vi "MultiDepth ILC Homing.vi"(7 "Offset Home 2 RCM":dbl[](array[numeric])=[0.0, 0.0, 0.0, 0.0], 8 "error in":errorcluster, 9 "Stage PID Cluster":T2={"Stage Z PID"={"Kp"=0.0005, "Kd"=0.001, "Ki"=0.0}, "Stage Y PID"={"Kp"=0.0003, "Kd"=0.01, "Ki"=0.0}, "Stage X PID"={"Kp"=0.0003, "Kd"=0.01, "Ki"=0.0}}, 10 "L1 to L4 PID Cluster":T1={"L1 PID Gains"={"Kp"=0.005, "Kd"=0.5, "Ki"=0.0005}, "L2 PID Gains"={"Kp"=0.01, "Kd"=1.0, "Ki"=0.005}, "L3 PID Gains"={"Kp"=0.05, "Kd"=1.0, "Ki"=0.0005}, "L4 PID Gains"={"Kp"=0.1, "Kd"=0.1, "Ki"=0.0005}}, 11 "FPGA VI Reference In":refnum<k20>) -> (0 "error out":errorcluster, 1 "Last Stage Posit":dbl[](array[numeric]), 2 "Last L1 to L4 Posit":dbl[](array[numeric]), 3 "FPGA VI Reference Out":refnum<k20>)   [LabVIEW 2016]
uses:
  <vilib>/Platform/TimedLoop/XDataNode/timing_clust.ctl
  <vilib>/Platform/TimedLoop/XDataNode/nitl_modes.ctl
  <vilib>/Platform/TimedLoop/XDataNode/wakeup.ctl
  Library/KevinLibraryAll/labview2010/kevLib2010/Simple Filters/kDelay.vi
  Global Variables.vi
  <vilib>/Utility/error.llb/Error Cluster From Error Code.vi
  <vilib>/rvi/errors/niLvFpgaAdjustHostInterfaceError.vi
  <vilib>/platform/TimedLoop/XDataNode/XDataNode.xnode
  <vilib>/rvi/interface/nirviReadWriteControl/nirviReadWriteControl.xnode
  FPGA Bitfiles/PhantomControlPI_FPGATarget_QuadCtr2_E2412E44.lvbitx
  IRISS_FPGA_IO.vi
  <vilib>/Platform/TimedLoop/XDataNode/XDNodeRunTimeDep.lvlib
  Library/KevinLibraryAll/labview2010/kevLib2010.lvlib
  Library/KevinLibraryAll/labview2011/kevLib2011.lvlib
  Library/KevinLibraryAll/labview/KevLib01.lvlib
  Library/jmslib.lvlib
  NiFpgaLv.dll
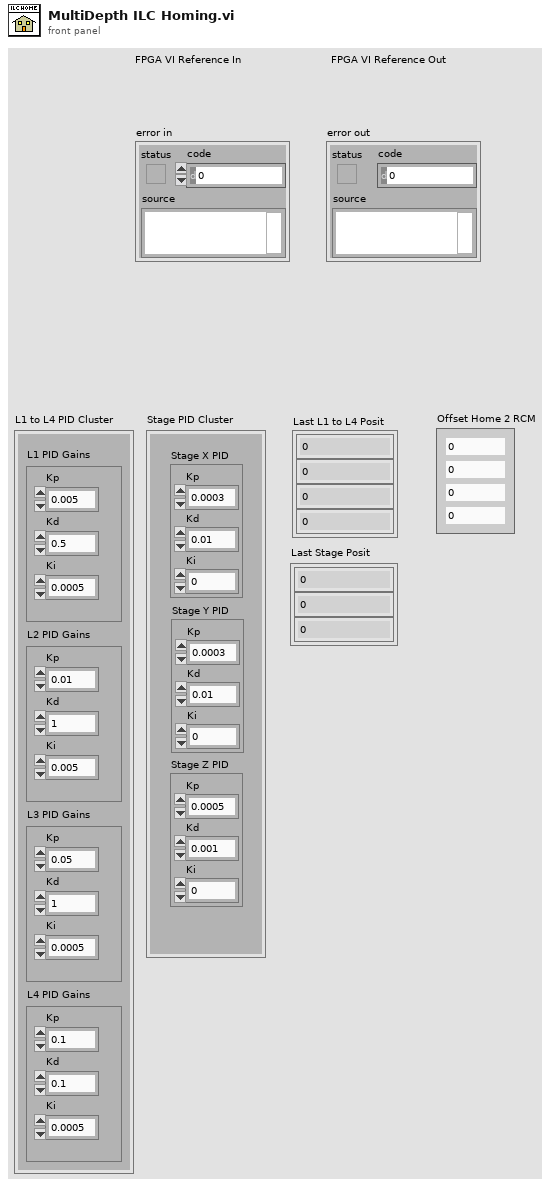
[diagram p1: front panel]
types:
  T1 = cluster{"L1 PID Gains":cluster{"Kp":dbl, "Kd":dbl, "Ki":dbl}, "L2 PID Gains":cluster{"Kp":dbl, "Kd":dbl, "Ki":dbl}, "L3 PID Gains":cluster{"Kp":dbl, "Kd":dbl, "Ki":dbl}, "L4 PID Gains":cluster{"Kp":dbl, "Kd":dbl, "Ki":dbl}}
  T2 = cluster{"Stage Z PID":cluster{"Kp":dbl, "Kd":dbl, "Ki":dbl}, "Stage Y PID":cluster{"Kp":dbl, "Kd":dbl, "Ki":dbl}, "Stage X PID":cluster{"Kp":dbl, "Kd":dbl, "Ki":dbl}}
  T3 = typedef "XDNodeRunTimeDep.lvlib/timing_clust.ctl" = cluster{"Expected End [f-1]":u64, "Actual End [f-1]":u64, "Finished Late? [f-1]":bool, "Expected End [i-1]":u64, "Actual End [i-1]":u64, "Finished Late? [i-1]":bool, "Expected Start [i]":u64, "Actual Start [i]":u64, "Expected Start [f]":u64, "Actual Start [f]":u64, "Source Name":string, "Structure Name":string, "Period":i64, "Deadline":i64, "Offset":i64, "Start":i64, "Priority":i32, "Timeout":i32, "Mode":T4, "Wakeup Reason":T5, "Error":errorcluster, "Source Type":string, "Secondary Source Type":string, "Global End Time":u64, "Global Start Time":u64, "Frame Duration":u64, "Iteration Duration":u64, "Assigned CPU":i32, "I/O Scan Engine Mode":u32}
  T4 = typedef "XDNodeRunTimeDep.lvlib/nitl_modes.ctl" = enum32{"No Change", "Process missed periods, maintain original phase", "Discard missed periods, maintain original phase", "Process missed periods, ignore original phase", "Discard missed periods, ignore original phase"}
  T5 = typedef "XDNodeRunTimeDep.lvlib/wakeup.ctl" = enum32{"Normal", "Aborted", "Asynchronous wakeup", "Timing source error", "Timed loop error", "Timeout"}
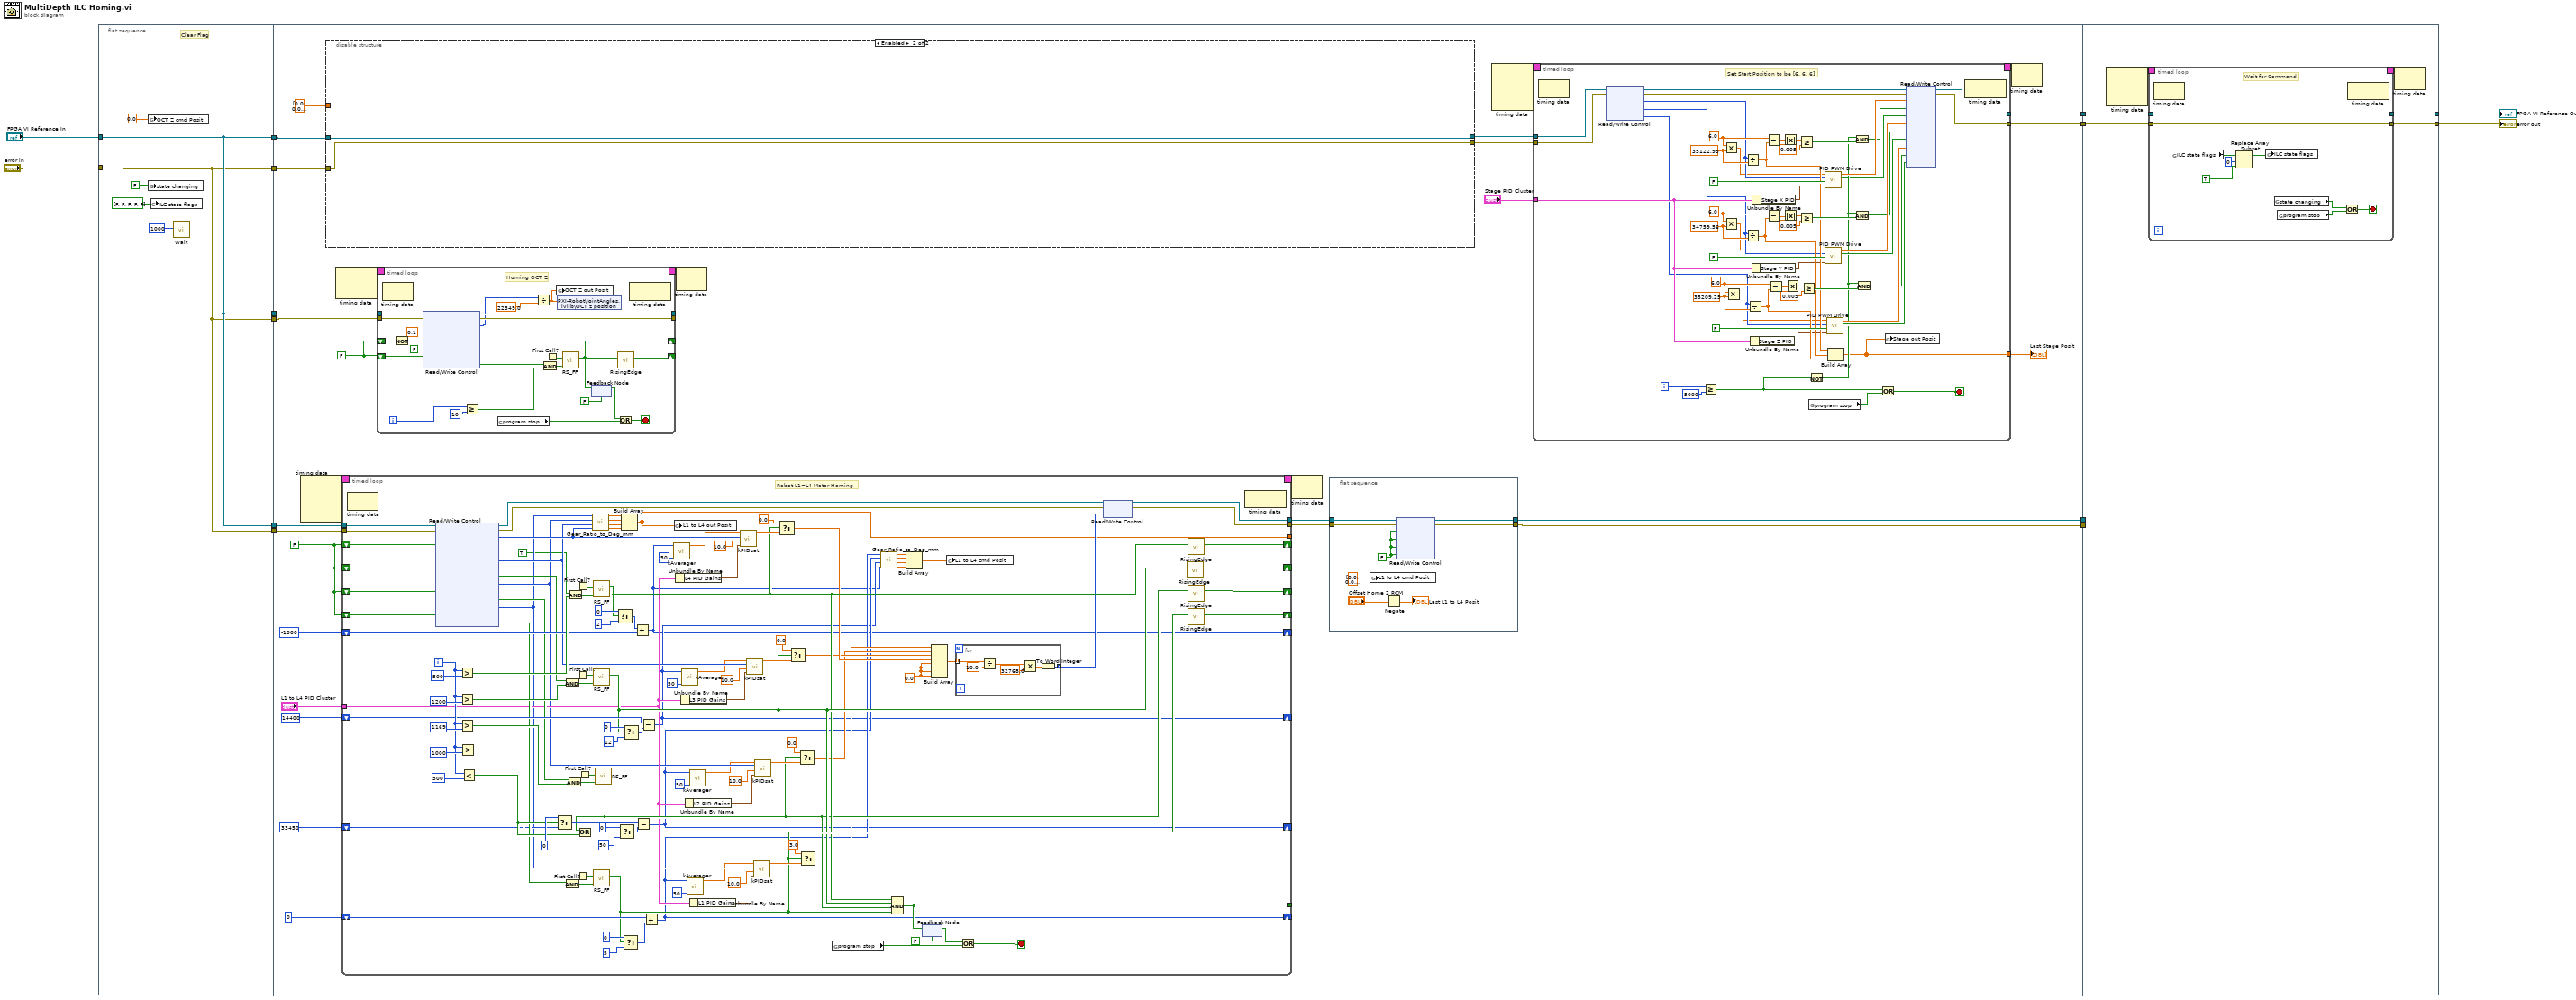
[diagram p0: block diagram]
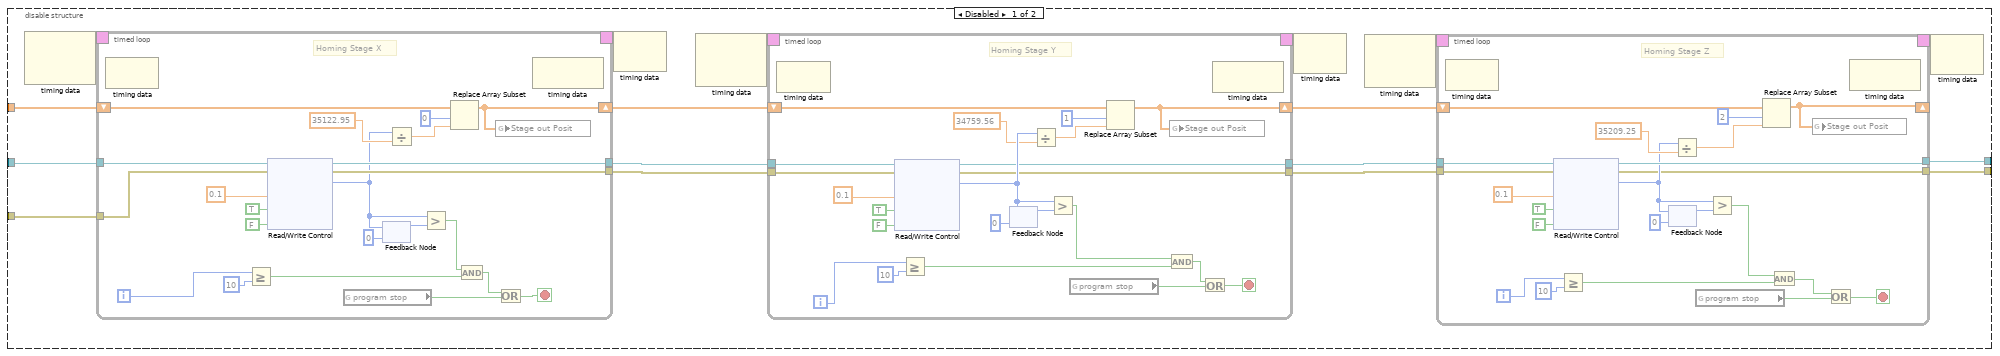
[diagram p2: hidden frame]
diagram:
  n1 = flat-sequence {
    tunnel: "FPGA VI Reference In" -> [w18]
    tunnel: "error in" -> [w17]
    tunnel: [w18] -> w14
    tunnel: [w18] -> w13
    tunnel: [w17] -> w12
    tunnel: [w17] -> w11
    tunnel: [w18] -> w6
    tunnel: [w17] -> w5
    tunnel: w14 -> [w48]
    tunnel: w13 -> [w47]
    tunnel: w12 -> [w46]
    tunnel: w11 -> [w45]
    tunnel: w6 -> [w42]
    tunnel: w5 -> [w41]
    tunnel: [w39] -> w4
    tunnel: [w38] -> w3
    tunnel: [w32] -> w2
    tunnel: [w31] -> w1
    tunnel: [w372] -> w8
    tunnel: [w371] -> w7
    tunnel: w4 -> [_]
    tunnel: w3 -> [_]
    tunnel: w2 -> [w370]
    tunnel: w1 -> [w369]
    frame #0 {
      # "Clear Flag"
      n2 = global write "Global Variables.vi" "OCT Z cmd Posit"(0.0) -> ()
      n3 = global write "Global Variables.vi" "state changing"(FALSE ("state changing")) -> ()
      n4 = global write "Global Variables.vi" "ILC state flags"(bool[] [FALSE, FALSE, FALSE, FALSE, FALSE]) -> ()
      n5 = call "Wait"("Count(mSec)"=u32 1000 ("milliseconds to wait")) -> ()  [unwired: 1 out]
    }
    frame #1 {
      w26 = FALSE ("Rising Edge")
      w40 = FALSE ("Rising Edge")
      n6 = node-c288() -> (w30:T3)  [unwired: 4 in]
      n7 = disable-structure shown="Enabled" {
        disable-tunnel: [w61 w147] -> w50
        disable-tunnel: [w60 w146] -> w49
        disable-tunnel: w48 -> [w59 w147]
        disable-tunnel: w46 -> [w58 w146]
        disable-tunnel: dbl[] [0.0, 0.0, 0.0] ("Stage Posit Array") -> [w51 _]
        frame Disabled {
          n8 = node-c288() -> (w63:T3)  [unwired: 2 in]
          n9 = timed-loop {
            timing: w63 -> [_]
            timing-out: [_] -> w62
            tunnel: w59 -> [w79]
            tunnel: w58 -> [w78]
            tunnel: [w77] -> w54
            tunnel: [w76] -> w53
            shift-right: [w68] -> w52
            shift-left: w51 -> [w70]
            i -> [w80]
            stop <- w73 stop-if-true
            # "Homing Stage X"
            n10 = node-c288() -> ()  [unwired: 1 in, 1 out]
            n11 = Greater Or Equal?(x=w80, y=10) -> (x >= y?=w89:bool)
            n12 = xnode "Read/Write Control"("FPGA VI Reference In"=w79, "error in"=w78, "X DC"=0.1 ("y"), "INHB X"=TRUE ("INHB Y"), "DIR X"=FALSE ("INHB Y")) -> ("FPGA VI Reference Out"=w77:refnum<k20>, "error out"=w76:errorcluster, "Position X"=w69:i32)
            n13 = global read "Global Variables.vi" "program stop"() -> (w75:bool)
            n14 = feedback #1(0 ("Position Y")) -> (w86:i32)
            n15 = feedback-in #1(w69) -> ()
            n16 = Divide(x=w69, y=35122.95) -> (x/y=w71:dbl)
            n17 = Greater?(x=w69, y=w86) -> (0:w87:bool)
            n18 = Replace Array Subset(array=w70, new element=w71, index=0) -> (w68:dbl[])
            n19 = And(x=w87, y=w89) -> (x .and. y?=w74:bool)
            n20 = global write "Global Variables.vi" "Stage out Posit"(w68) -> ()
            n21 = Or(x=w74, y=w75) -> (x .or. y?=w73:bool)
            n22 = node-c288() -> ()  [unwired: 1 in, 1 out]
          }
          n23 = node-c288(w62) -> ()  [unwired: 1 out]
          n24 = node-c288() -> (w65:T3)  [unwired: 2 in]
          n25 = timed-loop {
            timing: w65 -> [_]
            timing-out: [_] -> w64
            tunnel: w54 -> [w104]
            tunnel: w53 -> [w105]
            tunnel: [w102] -> w57
            tunnel: [w101] -> w56
            shift-right: [w94] -> w55
            shift-left: w52 -> [w95]
            i -> [w103]
            stop <- w100 stop-if-true
            # "Homing Stage Y"
            n26 = node-c288() -> ()  [unwired: 1 in, 1 out]
            n27 = xnode "Read/Write Control"("FPGA VI Reference In"=w104, "error in"=w105, "Y DC"=0.1 ("y"), "INHB Y"=TRUE, "DIR Y"=FALSE ("INHB Y")) -> ("FPGA VI Reference Out"=w102:refnum<k20>, "error out"=w101:errorcluster, "Position Y"=w112:i32)
            n28 = Greater Or Equal?(x=w103, y=10) -> (x >= y?=w115:bool)
            n29 = feedback #2(0 ("Position Y")) -> (w111:i32)
            n30 = feedback-in #2(w112) -> ()
            n31 = Divide(x=w112, y=34759.56) -> (x/y=w96:dbl)
            n32 = Greater?(x=w112, y=w111) -> (0:w113:bool)
            n33 = global read "Global Variables.vi" "program stop"() -> (w98:bool)
            n34 = Replace Array Subset(array=w95, new element=w96, index=1) -> (w94:dbl[])
            n35 = And(x=w113, y=w115) -> (x .and. y?=w99:bool)
            n36 = global write "Global Variables.vi" "Stage out Posit"(w94) -> ()
            n37 = Or(x=w99, y=w98) -> (x .or. y?=w100:bool)
            n38 = node-c288() -> ()  [unwired: 1 in, 1 out]
          }
          n39 = node-c288(w64) -> ()  [unwired: 1 out]
          n40 = node-c288() -> (w67:T3)  [unwired: 2 in]
          n41 = timed-loop {
            timing: w67 -> [_]
            timing-out: [_] -> w66
            tunnel: w57 -> [w141]
            tunnel: [w140] -> w61
            tunnel: w56 -> [w128]
            tunnel: [w127] -> w60
            shift-right: [w120] -> _
            shift-left: w55 -> [w121]
            i -> [w131]
            stop <- w125 stop-if-true
            # "Homing Stage Z"
            n42 = node-c288() -> ()  [unwired: 1 in, 1 out]
            n43 = xnode "Read/Write Control"("FPGA VI Reference In"=w141, "error in"=w128, "Z DC"=0.1 ("y"), "INHB Z"=TRUE ("INHB Y"), "DIR Z"=FALSE ("INHB Y")) -> ("FPGA VI Reference Out"=w140:refnum<k20>, "error out"=w127:errorcluster, "Position Z"=w133:i32)
            n44 = Greater Or Equal?(x=w131, y=10) -> (x >= y?=w129:bool)
            n45 = feedback-in #3(w133) -> ()
            n46 = feedback #3(0 ("Position Y")) -> (w134:i32)
            n47 = Divide(x=w133, y=35209.25) -> (x/y=w122:dbl)
            n48 = global read "Global Variables.vi" "program stop"() -> (w126:bool)
            n49 = Greater?(x=w133, y=w134) -> (0:w132:bool)
            n50 = Replace Array Subset(array=w121, new element=w122, index=2) -> (w120:dbl[])
            n51 = And(x=w132, y=w129) -> (x .and. y?=w124:bool)
            n52 = global write "Global Variables.vi" "Stage out Posit"(w120) -> ()
            n53 = Or(x=w124, y=w126) -> (x .or. y?=w125:bool)
            n54 = node-c288() -> ()  [unwired: 1 in, 1 out]
          }
          n55 = node-c288(w66) -> ()  [unwired: 1 out]
        }
        frame Enabled {
        }
      }
      n56 = node-c288() -> (w44:T3)  [unwired: 2 in]
      n57 = timed-loop {
        timing: w30 -> [_]
        timing-out: [_] -> w29
        tunnel: w47 -> [w262]
        tunnel: w45 -> [w261]
        shift-right: [w196] -> _
        shift-left: w26 -> [w260]
        shift-right: [w195] -> _
        shift-left: w26 -> [w259]
        shift-right: [w194] -> _
        shift-left: w26 -> [w258]
        shift-right: [w193] -> _
        shift-left: w26 -> [w257]
        shift-right: [w151] -> _
        shift-left: -1000 -> [w240]
        shift-right: [w152] -> _
        shift-left: 14400 -> [w232]
        shift-right: [w153] -> _
        shift-left: 33450 -> [w203]
        shift-right: [w154] -> _
        shift-left: 0 -> [w202]
        tunnel: [w197] -> _
        tunnel: [w177] -> w28
        tunnel: [w176] -> w27
        tunnel: "L1 to L4 PID Cluster" -> [w172]
        tunnel: [w150] -> _
        i -> [w242]
        stop <- w198 stop-if-true
        w188 = 0.0 ("element")
        # "Robot L1~L4 Motor Homing"
        n58 = node-c288() -> ()  [unwired: 1 in, 1 out]
        n59 = xnode "Read/Write Control"("FPGA VI Reference In"=w262, "error in"=w261, "Reset C1-4"=w260, "Reset C1-1"=w259, "Reset 3"=w258, "Reset 1"=w257) -> ("FPGA VI Reference Out"=w185:refnum<k20>, "error out"=w184:errorcluster, "32 bit Position C1-4"=w170:i32, "32 bit Position C1-1"=w169:i32, "Home L3"=w223:bool, "32 bit Position 3"=w168:i32, "Home L2"=w221:bool, "32 bit Position 1"=w167:i32, "Home L1"=w208:bool)  [unwired: 1 out]
        n60 = Greater?(x=w242, y=500) -> (0:w241:bool)
        n61 = Greater?(x=w242, y=1200) -> (0:w224:bool)
        n62 = Greater?(x=w242, y=1169) -> (0:w222:bool)
        n63 = Greater?(x=w242, y=1000) -> (0:w207:bool)
        n64 = Less?(x=w242, y=500) -> (x < y?=w214:bool)
        n65 = Select(t=0, s=w214, f=w203) -> (s? t:f=w219:i32)
        n66 = And(x=w223, y=w224) -> (x .and. y?=w233:bool)
        n67 = And(x=w208, y=w207) -> (x .and. y?=w209:bool)
        n68 = And(x=w221, y=w222) -> (x .and. y?=w226:bool)
        n69 = And(x=TRUE, y=w241) -> (x .and. y?=w253:bool)
        n70 = First Call?() -> (First Call?: T/F=w234:bool)
        n71 = First Call?() -> (First Call?: T/F=w210:bool)
        n72 = First Call?() -> (First Call?: T/F=w252:bool)
        n73 = First Call?() -> (First Call?: T/F=w225:bool)
        n74 = call "Gear_Ratio_to_Deg_mm.vi"("j4"=w170, "j3"=w169, "j2"=w168, "j1"=w167) -> ("theta 4"=w163:dbl, "theta 3"=w164:dbl, "theta 2"=w165:dbl, "theta 1"=w166:dbl)
        n75 = call "RS_FF.vi"("Set"=w253, "Reset"=w252) -> ("Result"=w190:bool)  [unwired: 9 in]
        n76 = call "RS_FF.vi"("Set"=w233, "Reset"=w234) -> ("Result"=w191:bool)  [unwired: 9 in]
        n77 = call "RS_FF.vi"("Set"=w209, "Reset"=w210) -> ("Result"=w192:bool)  [unwired: 9 in]
        n78 = call "RS_FF.vi"("Set"=w226, "Reset"=w225) -> ("Result"=w189:bool)  [unwired: 9 in]
        n79 = Or(x=w189, y=w214) -> (x .or. y?=w218:bool)
        n80 = Select(t=0, s=w190, f=2) -> (s? t:f=w254:i32)
        n81 = Select(t=0, s=w218, f=50) -> (s? t:f=w215:i32)
        n82 = Build Array(w166, w165, w164, w163) -> (w150:dbl[])
        n83 = Select(t=0, s=w192, f=5) -> (s? t:f=w213:i32)
        n84 = Select(t=0, s=w191, f=12) -> (s? t:f=w235:i32)
        n85 = Add(x=w254, y=w240) -> (x+y=w151:i32)
        n86 = Subtract(x=w219, y=w215) -> (x-y=w153:i32)
        n87 = Subtract(x=w232, y=w235) -> (x-y=w152:i32)
        n88 = Add(x=w202, y=w213) -> (x+y=w154:i32)
        n89 = call "kAverager.vi"("num avg"=50, "input"=w151) -> ("output"=w155:dbl)  [unwired: 9 in]
        n90 = global write "Global Variables.vi" "L1 to L4 out Posit"(w150) -> ()
        n91 = Unbundle By Name(w172) -> ("L4 PID Gains"=w175:cluster{"Kp":dbl, "Kd":dbl, "Ki":dbl})
        n92 = Unbundle By Name(w172) -> ("L3 PID Gains"=w174:cluster{"Kp":dbl, "Kd":dbl, "Ki":dbl})
        n93 = call "kAverager.vi"("num avg"=50, "input"=w152) -> ("output"=w156:dbl)  [unwired: 9 in]
        n94 = Unbundle By Name(w172) -> ("L2 PID Gains"=w173:cluster{"Kp":dbl, "Kd":dbl, "Ki":dbl})
        n95 = call "kAverager.vi"("num avg"=50, "input"=w154) -> ("output"=w158:dbl)  [unwired: 9 in]
        n96 = call "kAverager.vi"("num avg"=50, "input"=w153) -> ("output"=w157:dbl)  [unwired: 9 in]
        n97 = Unbundle By Name(w172) -> ("L1 PID Gains"=w171:cluster{"Kp":dbl, "Kd":dbl, "Ki":dbl})
        n98 = call "kPIDsat.vi"("PID Gains"=w175, "Sat Limit"=10.0, "Position"=w170, "Reference"=w155) -> ("Control"=w249:dbl)  [unwired: 7 in]
        n99 = call "kPIDsat.vi"("PID Gains"=w174, "Sat Limit"=10.0, "Position"=w169, "Reference"=w156) -> ("Control"=w230:dbl)  [unwired: 7 in]
        n100 = call "kPIDsat.vi"("PID Gains"=w171, "Sat Limit"=10.0, "Position"=w167, "Reference"=w158) -> ("Control"=w204:dbl)  [unwired: 7 in]
        n101 = call "kPIDsat.vi"("PID Gains"=w173, "Sat Limit"=10.0, "Position"=w168, "Reference"=w157) -> ("Control"=w229:dbl)  [unwired: 7 in]
        n102 = Select(t=0.0, s=w190, f=w249) -> (s? t:f=w183:dbl)
        n103 = Select(t=0.0 ("element"), s=w191, f=w230) -> (s? t:f=w182:dbl)
        n104 = Select(t=0.0 ("element"), s=w189, f=w229) -> (s? t:f=w181:dbl)
        n105 = Select(t=3.0 ("element"), s=w192, f=w204) -> (s? t:f=w180:dbl)
        n106 = global read "Global Variables.vi" "program stop"() -> (w199:bool)
        n107 = call "Gear_Ratio_to_Deg_mm.vi"("j4"=w151, "j3"=w152, "j2"=w153, "j1"=w154) -> ("theta 4"=w159:dbl, "theta 3"=w160:dbl, "theta 2"=w161:dbl, "theta 1"=w162:dbl)
        n108 = Compound Arithmetic op=AND(w190, w191, w189, w192) -> (w197:bool)
        n109 = Build Array(w162, w161, w160, w159) -> (w149:dbl[])
        n110 = feedback #4(FALSE) -> (w200:bool)
        n111 = feedback-in #4(w197) -> ()
        n112 = Build Array(w180, w181, w182, w183, w188, w188, w188, w188) -> (w187:dbl[])
        n113 = global write "Global Variables.vi" "L1 to L4 cmd Posit"(w149) -> ()
        n114 = for {
          tunnel: [w266] -> w186 mode=indexing
          tunnel: w187 -> [w265] mode=indexing
          n115 = Divide(x=w265, y=10.0) -> (x/y=w268:dbl)
          n116 = Multiply(x=w268, y=32768.0) -> (x*y=w267:dbl)
          n117 = To Word Integer(number=w267) -> (16bit integer=w266:i16)
        }
        n118 = Or(x=w200, y=w199) -> (x .or. y?=w198:bool)
        n119 = xnode "Read/Write Control"("FPGA VI Reference In"=w185, "error in"=w184, "AO"=w186) -> ("FPGA VI Reference Out"=w177:refnum<k20>, "error out"=w176:errorcluster)
        n120 = call "RisingEdge.vi"("Signal In"=w191) -> ("Rising Edge"=w195:bool)  [unwired: 10 in]
        n121 = call "RisingEdge.vi"("Signal In"=w190) -> ("Rising Edge"=w196:bool)  [unwired: 10 in]
        n122 = call "RisingEdge.vi"("Signal In"=w189) -> ("Rising Edge"=w194:bool)  [unwired: 10 in]
        n123 = call "RisingEdge.vi"("Signal In"=w192) -> ("Rising Edge"=w193:bool)  [unwired: 10 in]
        n124 = node-c288() -> ()  [unwired: 1 in, 1 out]
      }
      n125 = timed-loop {
        timing: w44 -> [_]
        timing-out: [_] -> w43
        tunnel: w42 -> [w360]
        tunnel: w41 -> [w359]
        tunnel: [w358] -> _
        tunnel: [w357] -> _
        shift-right: [w352] -> _
        shift-left: w40 -> [w354]
        shift-right: [w348] -> _
        shift-left: w40 -> [w346]
        i -> [w361]
        stop <- w355 stop-if-true
        # "Homing OCT Z"
        n126 = node-c288() -> ()  [unwired: 1 in, 1 out]
        n127 = Not(x=w346) -> (.not. x?=w345:bool)
        n128 = xnode "Read/Write Control"("FPGA VI Reference In"=w360, "error in"=w359, "OCT Mot DC"=0.1 ("y"), "INHB OCT Mot"=w345, "DIR OCT Mot"=FALSE ("INHB Y"), "Reset 14"=w354) -> ("FPGA VI Reference Out"=w358:refnum<k20>, "error out"=w357:errorcluster, "32 bit Position 14"=w343:i32, "Home OCT z"=w353:bool)
        n129 = Greater Or Equal?(x=w361, y=10) -> (x >= y?=w364:bool)
        n130 = global read "Global Variables.vi" "program stop"() -> (w356:bool)
        n131 = Divide(x=w343, y=22349.0) -> (x/y=w341:dbl)
        n132 = And(x=w353, y=w364) -> (x .and. y?=w350:bool)
        n133 = First Call?() -> (First Call?: T/F=w351:bool)
        n134 = global write "Global Variables.vi" "OCT Z out Posit"(w341) -> ()
        n135 = shared-variable "PXI-Robot\\JointAngles.lvlib\\OCT z position"(w341) -> ()  [unwired: 1 in, 1 out]
        n136 = call "RS_FF.vi"("Set"=w350, "Reset"=w351) -> ("Result"=w348:bool)  [unwired: 9 in]
        n137 = feedback #5(FALSE) -> (w347:bool)
        n138 = feedback-in #5(w348) -> ()
        n139 = call "RisingEdge.vi"("Signal In"=w348) -> ("Rising Edge"=w352:bool)  [unwired: 10 in]
        n140 = Or(x=w347, y=w356) -> (x .or. y?=w355:bool)
        n141 = node-c288() -> ()  [unwired: 1 in, 1 out]
      }
      n142 = node-c288(w43) -> ()  [unwired: 1 out]
      n143 = node-c288(w29) -> ()  [unwired: 1 out]
      n144 = flat-sequence {
        tunnel: w28 -> [w279]
        tunnel: w27 -> [w278]
        tunnel: [w274] -> w39
        tunnel: [w273] -> w38
        frame #0 {
          w280 = FALSE ("Reset 1")
          n145 = global write "Global Variables.vi" "L1 to L4 cmd Posit"(dbl[] [0.0, 0.0, 0.0, 0.0] ("L1 to L4 cmd Posit")) -> ()
          n146 = Negate(x="Offset Home 2 RCM") -> (-x=→"Last L1 to L4 Posit":dbl[])
          n147 = xnode "Read/Write Control"("FPGA VI Reference In"=w279, "error in"=w278, "Reset C1-4"=w280, "Reset C1-1"=w280, "Reset 3"=w280, "Reset 1"=w280) -> ("FPGA VI Reference Out"=w274:refnum<k20>, "error out"=w273:errorcluster)
        }
      }
      n148 = node-c288() -> (w37:T3)  [unwired: 4 in]
      n149 = timed-loop {
        timing: w37 -> [_]
        timing-out: [_] -> w36
        tunnel: w50 -> [w301]
        tunnel: w49 -> [w302]
        tunnel: "Stage PID Cluster" -> [w310]
        tunnel: [w283] -> w34
        tunnel: [w282] -> w32
        tunnel: [w281] -> w31
        i -> [w336]
        stop <- w300 stop-if-true
        w313 = 6.0 ("y")
        w316 = 35209.25 ("y")
        w327 = 6.0 ("y")
        w324 = 34759.56 ("y")
        w328 = 6.0 ("y")
        w331 = 35122.95 ("y")
        # "Set Start Position to be [6, 6, 6]"
        n150 = node-c288() -> ()  [unwired: 1 in, 1 out]
        n151 = xnode "Read/Write Control"("FPGA VI Reference In"=w301, "error in"=w302) -> ("FPGA VI Reference Out"=w304:refnum<k20>, "error out"=w303:errorcluster, "Position X"=w299:i32, "Position Y"=w298:i32, "Position Z"=w297:i32)
        n152 = Greater Or Equal?(x=w336, y=5000) -> (x >= y?=w289:bool)
        n153 = Multiply(x=w328, y=w331) -> (x*y=w296:dbl)
        n154 = Multiply(x=w327, y=w324) -> (x*y=w295:dbl)
        n155 = Multiply(x=w313, y=w316) -> (x*y=w294:dbl)
        n156 = Divide(x=w299, y=w331) -> (x/y=w309:dbl)
        n157 = Divide(x=w298, y=w324) -> (x/y=w308:dbl)
        n158 = Divide(x=w297, y=w316) -> (x/y=w307:dbl)
        n159 = Unbundle By Name(w310) -> ("Stage Z PID"=w305:cluster{"Kp":dbl, "Kd":dbl, "Ki":dbl})
        n160 = Unbundle By Name(w310) -> ("Stage Y PID"=w306:cluster{"Kp":dbl, "Kd":dbl, "Ki":dbl})
        n161 = Unbundle By Name(w310) -> ("Stage X PID"=w290:cluster{"Kp":dbl, "Kd":dbl, "Ki":dbl})
        n162 = Subtract(x=w328, y=w309) -> (x-y=w332:dbl)
        n163 = Subtract(x=w327, y=w308) -> (x-y=w323:dbl)
        n164 = Subtract(x=w313, y=w307) -> (x-y=w317:dbl)
        n165 = Absolute Value(x=w332) -> (abs(x)=w333:dbl)
        n166 = Absolute Value(x=w323) -> (abs(x)=w322:dbl)
        n167 = Absolute Value(x=w317) -> (abs(x)=w318:dbl)
        n168 = Greater Or Equal?(x=w333, y=0.005) -> (x >= y?=w329:bool)
        n169 = Greater Or Equal?(x=w322, y=0.005) -> (x >= y?=w326:bool)
        n170 = Greater Or Equal?(x=w318, y=0.005) -> (x >= y?=w314:bool)
        n171 = Not(x=w289) -> (.not. x?=w288:bool)
        n172 = global read "Global Variables.vi" "program stop"() -> (w311:bool)
        n173 = call "PID PWM Drive.vi"("PID Gains"=w290, "Reverse Motor?"=FALSE, "Encoder Position"=w299, "Reference"=w296) -> ("Direction"=w286:bool, "Duty Cycle"=w293:dbl)  [unwired: 5 in, 1 out]
        n174 = call "PID PWM Drive.vi"("PID Gains"=w306, "Reverse Motor?"=FALSE, "Encoder Position"=w298, "Reference"=w295) -> ("Direction"=w320:bool, "Duty Cycle"=w292:dbl)  [unwired: 5 in, 1 out]
        n175 = call "PID PWM Drive.vi"("PID Gains"=w305, "Reverse Motor?"=FALSE, "Encoder Position"=w297, "Reference"=w294) -> ("Direction"=w312:bool, "Duty Cycle"=w291:dbl)  [unwired: 5 in, 1 out]
        n176 = Build Array(w309, w308, w307) -> (w283:dbl[])
        n177 = And(x=w288, y=w329) -> (x .and. y?=w287:bool)
        n178 = And(x=w288, y=w326) -> (x .and. y?=w285:bool)
        n179 = And(x=w288, y=w314) -> (x .and. y?=w284:bool)
        n180 = Or(x=w289, y=w311) -> (x .or. y?=w300:bool)
        n181 = global write "Global Variables.vi" "Stage out Posit"(w283) -> ()
        n182 = xnode "Read/Write Control"("FPGA VI Reference In"=w304, "error in"=w303, "X DC"=w293, "INHB X"=w287, "DIR X"=w286, "Y DC"=w292, "INHB Y"=w285, "DIR Y"=w320, "Z DC"=w291, "INHB Z"=w284, "DIR Z"=w312) -> ("FPGA VI Reference Out"=w282:refnum<k20>, "error out"=w281:errorcluster)
        n183 = node-c288() -> ()  [unwired: 1 in, 1 out]
      }
      "Last Stage Posit" <- w34
      n184 = node-c288(w36) -> ()  [unwired: 1 out]
    }
    frame #2 {
      n185 = node-c288() -> (w374:T3)  [unwired: 3 in]
      n186 = timed-loop {
        timing: w374 -> [_]
        timing-out: [_] -> w373
        tunnel: w370 -> [w377]
        tunnel: [w377] -> w372
        tunnel: [w376] -> w371
        tunnel: w369 -> [w376]
        stop <- w375 stop-if-true
        # "Wait for Command"
        n187 = node-c288() -> ()  [unwired: 1 in, 1 out]
        n188 = global read "Global Variables.vi" "ILC state flags"() -> (w381:bool[])
        n189 = Replace Array Subset(array=w381, new element=TRUE ("new element/subarray"), index=0) -> (w380:bool[])
        n190 = global write "Global Variables.vi" "ILC state flags"(w380) -> ()
        n191 = global read "Global Variables.vi" "state changing"() -> (w383:bool)
        n192 = global read "Global Variables.vi" "program stop"() -> (w382:bool)
        n193 = Or(x=w383, y=w382) -> (x .or. y?=w375:bool)
        n194 = node-c288() -> ()  [unwired: 1 in, 1 out]
      }
      n195 = node-c288(w373) -> ()  [unwired: 1 out]
    }
  }
  "FPGA VI Reference Out" <- w8
  "error out" <- w7
